vi "Init.vi"(8 "error in (no error)":errorcluster) -> (0 "error out":errorcluster, 3 "Robot_Interface out":refnum<class "Robot_Interface.lvclass">)   [LabVIEW 2015, in "Robot_Interface.lvclass"]
uses:
  Robot_Interface.lvclass
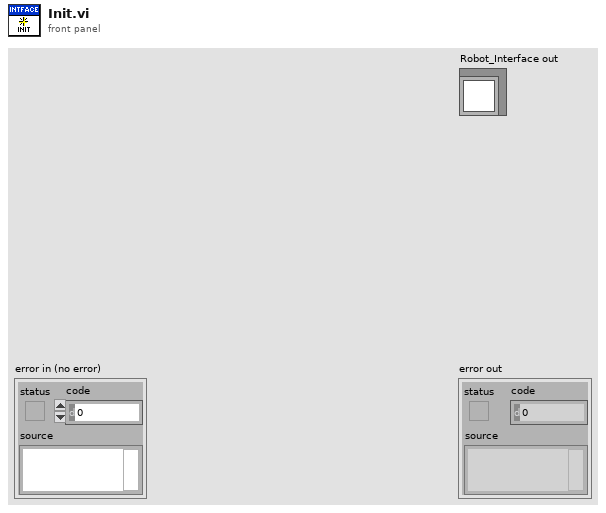
[diagram p1: front panel]
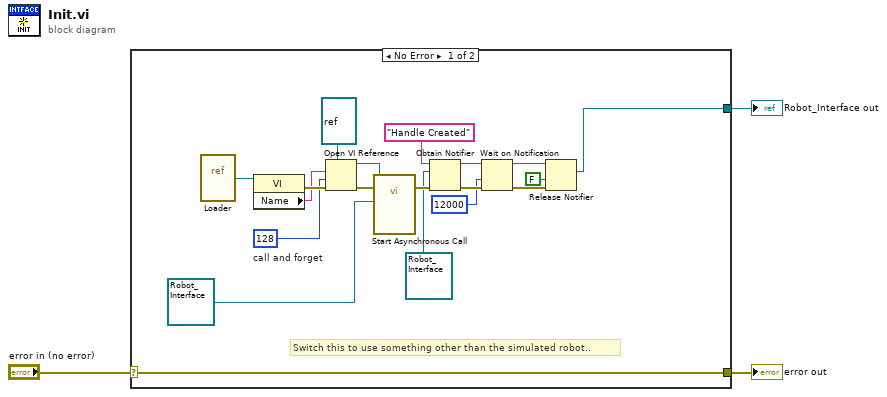
[diagram p0: block diagram]
diagram:
  n1 = case shown="No Error" "error in (no error)" {
    selector: "error in (no error)" -> [w22 w23]
    tunnel: [w22 w23] -> w2
    tunnel: [w5 _] -> w1
    frame No Error {
      w16 = 128  # call and forget
      # "Switch this to use something other than the simulated robot.."
      n2 = vi-ref "Loader.vi"() -> (w20:refnum<vi>)
      n3 = property class="VI"(reference=w20) -> (error out=w19:errorcluster, "Name"=w17:string)  [unwired: 1 in, 1 out]
      n4 = Open VI Reference(type specifier VI Refnum (for type only)=refnum<vi> refnum, vi path=w17, options=w16, error in (no error)=w19) -> (vi reference=w14:refnum<vi>, error out=w15:errorcluster)  [unwired: 2 in]
      n5 = call-by-ref "Start Asynchronous Call"(reference=w14, error in=w15, "Robot_Interface"=refnum<class "Robot_Interface.lvclass"> refnum (".NET_Robot_Interface.lvclass")) -> (error out=w13:errorcluster)  [unwired: 11 in, 1 out]
      n6 = Obtain Notifier(name (unnamed)="Handle Created", notification data type=refnum<class "Robot_Interface.lvclass"> refnum ("Robot_Interface in"), error in (no error)=w13) -> (notifier out=w12:refnum<notifier>, error out=w11:errorcluster)  [unwired: 1 in, 1 out]
      n7 = Wait on Notification(notifier=w12, timeout in ms (-1)=12000, error in (no error)=w11) -> (notifier out=w9:refnum<notifier>, error out=w8:errorcluster)  [unwired: 1 in, 2 out]
      n8 = Release Notifier(notifier=w9, force destroy? (F)=FALSE, error in (no error)=w8) -> (last notification=w5:refnum<class "Robot_Interface.lvclass">)  [unwired: 2 out]
    }
    frame Error {
    }
  }
  "error out" <- w2
  "Robot_Interface out" <- w1
